vi "Write Low Alarm Limit.vi"(8 "error in":errorcluster, 10 "low alarm limit":dbl format="%.2f", 11 "Has Alarm Limits in":refnum<class "Has Alarm Limits.lvclass">) -> (0 "error out":errorcluster, 3 "Has Alarm Limits out":refnum<class "Has Alarm Limits.lvclass">)   [LabVIEW 2020, in "PV Access.lvlib" / "PV Data.lvlib" / "Has Alarm Limits.lvclass"]
uses:
  Has Alarm Limits.lvclass
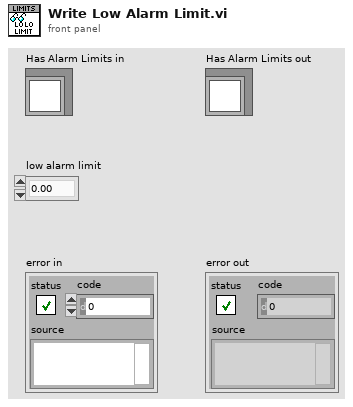
[diagram p1: front panel]
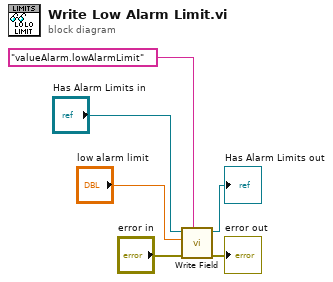
[diagram p0: block diagram]
diagram:
  n1 = call-dynamic "Write Field.vi"("field"="valueAlarm.lowAlarmLimit" ("element name"), "error in (no error)"="error in", "value"="low alarm limit", "Base Interface in"="Has Alarm Limits in") -> ("error out"=→"error out":errorcluster, "Base Interface out"=→"Has Alarm Limits out":refnum<class "Has Alarm Limits.lvclass">)  [unwired: 6 in]
